vi "Destroy.vi"(8 "error in (no error)":errorcluster, 11 "logger in":refnum<class "Logger.lvclass">) -> (0 "error out":errorcluster, 3 "failure info":T1 {"Log Record"."timestamp" format="%<%x %.3X>T"})   [LabVIEW 2024, in "Logging.lvlib" / "Logger.lvclass"]
uses:
  Logger.lvclass
  Failure Information.ctl
  Log Record.ctl
  Internal Log Levels.ctl
  Logger.lvclass/Logger.ctl
  Handlers/Formatting Handler/Formatting Handler.lvclass
  Logging.lvlib
panel:
  # "Connector Pane"
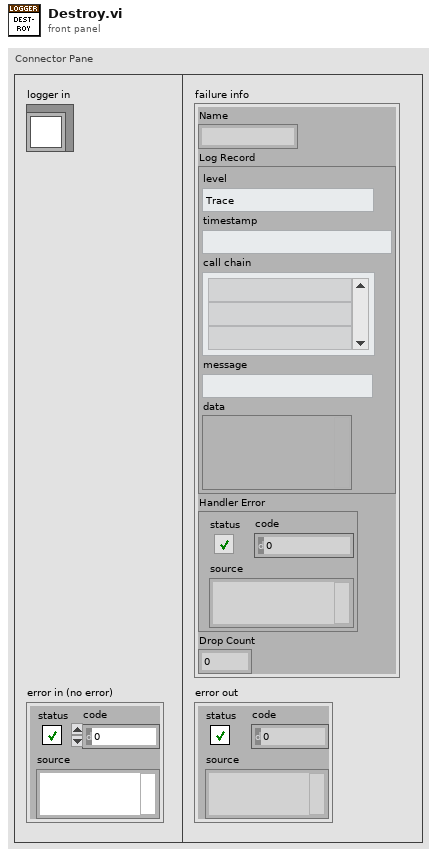
[diagram p1: front panel]
types:
  T1 = typedef "Failure Information.ctl" = cluster{"Name":string, "Log Record":T2, "Handler Error":errorcluster, "Drop Count":u32}
  T2 = typedef "Logging.lvlib/Log Record.ctl" = cluster{"level":T3, "timestamp":timestamp, "call chain":string[], "message":string, "data":variant}
  T3 = typedef "Logging.lvlib/Internal Log Levels.ctl" = enum16{"Trace", "Debug", "Info", "Warning", "Error", "Critical", "Internal"}
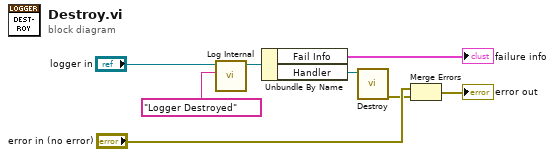
[diagram p0: block diagram]
diagram:
  n1 = call "Log Internal.vi"("message"="Logger Destroyed", "logger in"="logger in") -> ("logger out"=w4:refnum<class "Logger.lvclass">)  [unwired: 9 in]
  n2 = Unbundle By Name(w4) -> ("Fail Info"=→"failure info":T1, "Handler"=w8:refnum<class "Formatting Handler.lvclass">)
  n3 = call-dynamic "Destroy.vi"("handler in"=w8) -> ("error out"=w6:errorcluster)  [unwired: 10 in]
  n4 = Merge Errors("error in (no error)", w6) -> (→"error out":errorcluster)
